vi "nntcp.vi"() -> ()   [LabVIEW 2018, in "nn.lvlib"]
uses:
  nn.lvlib
panel:
  out "resulting string 2":string
  out "data out 2":string
  in  "Train":bool=TRUE
  out "Waveform Output":dbl
  out "Class Indicator":i32
  in  "Waveform Selection":enum16{"Sine", "Square", "Triangle", "Sawtooth"}(ring)
  out "Signal":dynamicdata(graph) caption="Sine"
  in  "Port":u16=54321
  out "error out":errorcluster
  in  "Stop Button":bool
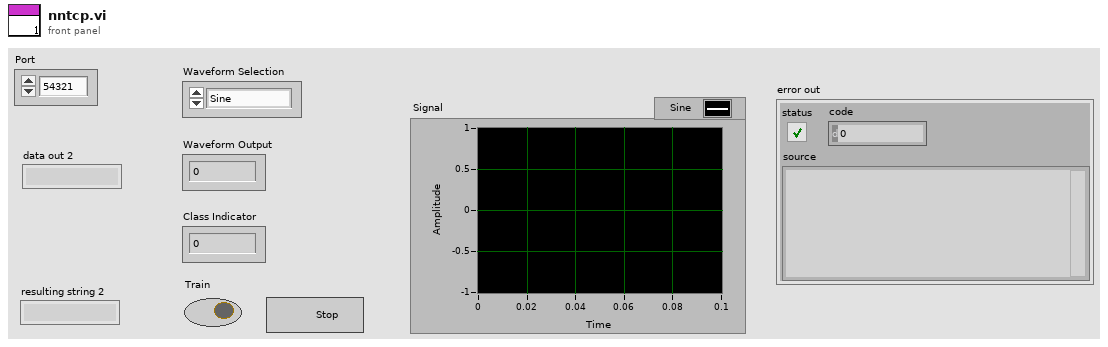
[diagram p1: front panel]
types:
  T1 = enum16{"Standard", "Buffered", "CRLF", "Immediate"}
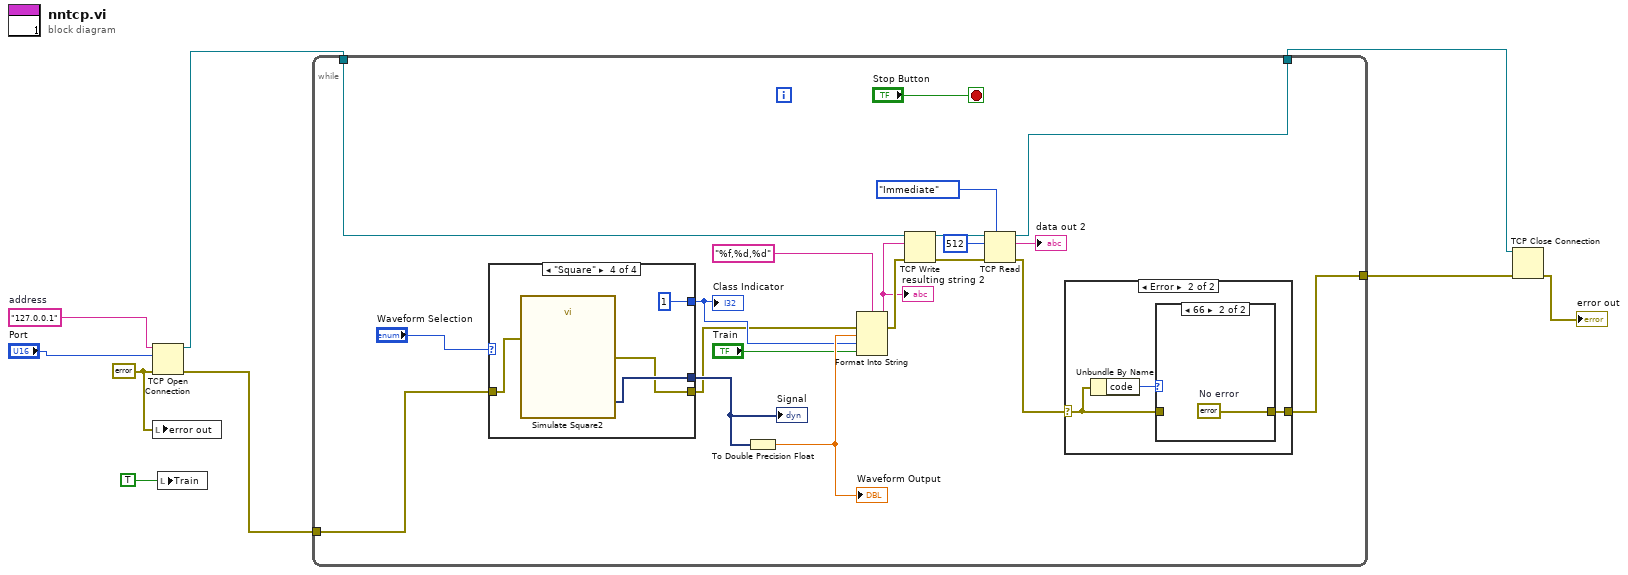
[diagram p0: block diagram]
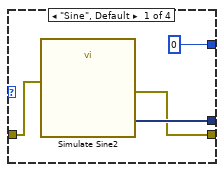
[diagram p4: hidden frame]
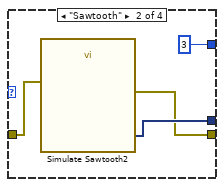
[diagram p5: hidden frame]
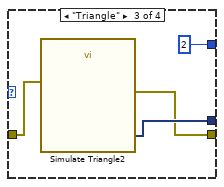
[diagram p6: hidden frame]
diagram:
  w6 = errorcluster {"status"=FALSE, "code"=0, "source"=""} ("error in (no error)")
  w9 = "127.0.0.1"  # address
  n1 = TCP Open Connection(address=w9, remote port or service name="Port", error in (no error)=w6) -> (connection ID=w3:refnum<k5>, error out=w5:errorcluster)  [unwired: 2 in]
  n2 = local write "error out"(w6) -> ()
  n3 = local write "Train"(TRUE ("Train 2")) -> ()
  n4 = while {
    tunnel: w5 -> [w13]
    tunnel: [w12] -> w4
    tunnel: w3 -> [w11]
    tunnel: [w10] -> w2
    stop <- "Stop Button" stop-if-true
    n5 = case shown="\"Square\"" "Waveform Selection" {
      tunnel: [w39 w43 w47 w51] -> w27
      tunnel: [0 ("Numeric Indicator") 3 ("Numeric Indicator") 2 ("Numeric Indicator") 1 ("Numeric Indicator")] -> w19
      tunnel: [w37 w41 w45 w49] -> w18
      tunnel: w13 -> [w36 w40 w44 w48]
      frame "Sine", Default {
        n6 = call "Simulate Sine2"("error in (no error)"=w36) -> ("Sine"=w39:dynamicdata, "error out"=w37:errorcluster)  [unwired: 13 in]
      }
      frame "Sawtooth" {
        n7 = call "Simulate Sawtooth2"("error in (no error)"=w40) -> ("Sawtooth"=w43:dynamicdata, "error out"=w41:errorcluster)  [unwired: 13 in]
      }
      frame "Triangle" {
        n8 = call "Simulate Triangle2"("error in (no error)"=w44) -> ("Triangle"=w47:dynamicdata, "error out"=w45:errorcluster)  [unwired: 13 in]
      }
      frame "Square" {
        n9 = call "Simulate Square2"("error in (no error)"=w48) -> ("Square"=w51:dynamicdata, "error out"=w49:errorcluster)  [unwired: 13 in]
      }
    }
    "Signal" <- w27
    "Class Indicator" <- w19
    n10 = To Double Precision Float(number=w27) -> (double precision float=w21:dbl)
    "Waveform Output" <- w21
    n11 = Format Into String(format string="%f,%d,%d", error in=w18, w21, w19, "Train") -> (resulting string=w16:string, error out=w17:errorcluster)  [unwired: 1 in]
    "resulting string 2" <- w16
    n12 = TCP Write(connection ID=w11, data in=w16, error in (no error)=w17) -> (connection ID out=w25:refnum<k5>, error out=w26:errorcluster)  [unwired: 1 in, 1 out]
    n13 = TCP Read(connection ID=w25, bytes to read=512, error in (no error)=w26, 7:T1."Immediate" ("mode (standard)")) -> (connection ID out=w10:refnum<k5>, data out=→"data out 2":string, error out=w15:errorcluster)  [unwired: 1 in]
    n14 = case shown="Error" w15 {
      selector: w15 -> [w30 w32]
      tunnel: [w30 w31] -> w12
      frame No Error {
      }
      frame Error {
        n15 = Unbundle By Name(w32) -> ("code"=w33:i32)
        n16 = case shown="66" w33 {
          tunnel: w32 -> [w34 _]
          tunnel: [w34 w35] -> w31
          frame Default {
          }
          frame 66 {
            w35 = errorcluster {"status"=FALSE, "code"=0, "source"=""}  # No error
          }
        }
      }
    }
  }
  n17 = TCP Close Connection(connection ID=w2, error in (no error)=w4) -> (error out=→"error out":errorcluster)  [unwired: 1 in, 1 out]
